vi "Up-Down Control.vi"(8 "error in (no error)":errorcluster, 10 "Selection":i32, 11 "DataGrid Config Dialog in":refnum<class "DataGrid Config Dialog.lvclass">) -> (0 "error out":errorcluster, 3 "DataGrid Config Dialog out":refnum<class "DataGrid Config Dialog.lvclass">)   [LabVIEW 2018, in "DataGrid Config Dialog.lvclass"]
uses:
  DataGrid Config Dialog.lvclass
  DataGrid Config Dialog.lvclass/DataGrid Config Dialog.ctl
  DataGrid Config/DataGrid Config.lvclass
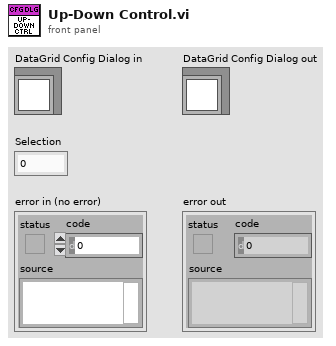
[diagram p1: front panel]
types:
  T1 = enum8{"Enabled", "Disabled", "Disabled and Grayed Out"}
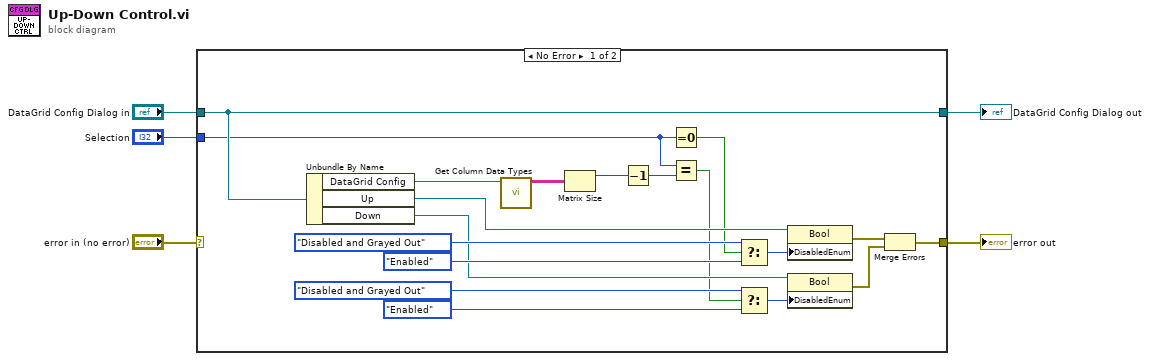
[diagram p0: block diagram]
diagram:
  n1 = case shown="No Error" "error in (no error)" {
    selector: "error in (no error)" -> [_ w26]
    tunnel: [w8 w26] -> w4
    tunnel: [w24 w25] -> w2
    tunnel: "DataGrid Config Dialog in" -> [w24 w25]
    tunnel: "Selection" -> [w21 _]
    frame No Error {
      n2 = Unbundle By Name(w24) -> ("DataGrid Config"=w7:refnum<class "DataGrid Config.lvclass">, "Up"=w20:refnum<vi>, "Down"=w15:refnum<vi>)
      n3 = call "Get Column Data Types.vi"("DataGrid Config"=w7) -> ("Column Data Type Names"=w6:string[][])  [unwired: 10 in]
      n4 = Matrix Size(0:w6) -> (1:w23:i32)  [unwired: 1 out]
      n5 = Decrement(x=w23) -> (x-1=w22:i32)
      n6 = Equal To 0?(x=w21) -> (x = 0?=w16:bool)
      n7 = Equal?(x=w21, y=w22) -> (x = y?=w12:bool)
      n8 = Select(t=T1."Disabled and Grayed Out" ("Disabled"), s=w16, f=T1."Enabled" ("Disabled")) -> (s? t:f=w17:T1)
      n9 = Select(t=T1."Disabled and Grayed Out" ("Disabled"), s=w12, f=T1."Enabled" ("Disabled")) -> (s? t:f=w11:T1)
      n10 = property class="Bool"(reference=w20, "DisabledEnum"=w17) -> (error out=w10:errorcluster)  [unwired: 1 in, 1 out]
      n11 = property class="Bool"(reference=w15, "DisabledEnum"=w11) -> (error out=w9:errorcluster)  [unwired: 1 in, 1 out]
      n12 = Merge Errors(w10, w9) -> (w8:errorcluster)
    }
    frame Error {
    }
  }
  "error out" <- w4
  "DataGrid Config Dialog out" <- w2
